vi "Debug Messages.vi"() -> ()   [LabVIEW 2021, in "YActor.lvclass"]
uses:
  YActor.lvclass
panel:
  in  "Debug Messages":cluster{"Msg":string, "Active":bool}[](array[cluster])
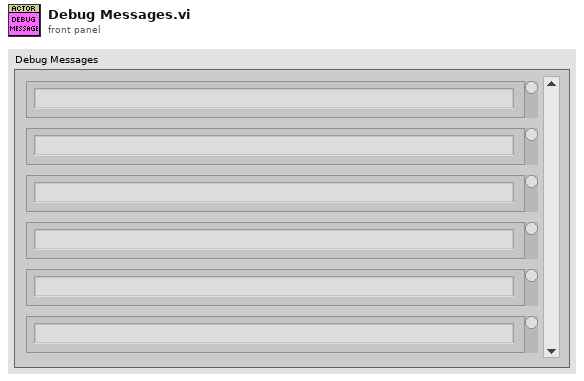
[diagram p1: front panel]
diagram:
